vi "有符号24位转32位有符号数.vi"(11 "Registers":u16[](array[numeric])) -> (2 "数字量":i32[](array[numeric]), 3 "工程量":dbl[](array[numeric]))   [LabVIEW 2016, in "采配水.lvlib"]
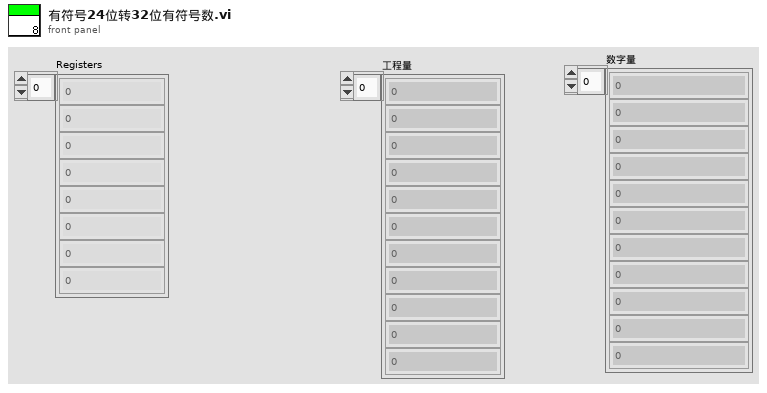
[diagram p1: front panel]
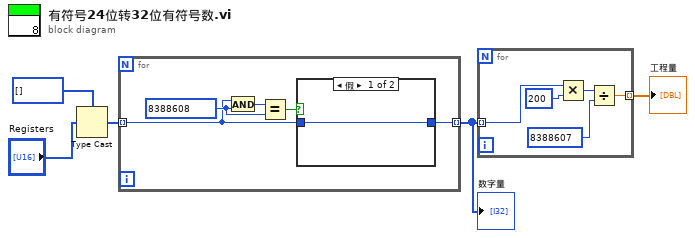
[diagram p0: block diagram]
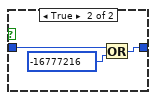
[diagram p2: hidden frame]
diagram:
  n1 = Type Cast(type=i32[] [], x="Registers") -> (*(type *) &x=w3:i32[])
  n2 = for {
    tunnel: w3 -> [w7] mode=indexing
    tunnel: [w6] -> w2 mode=indexing
    w9 = 8388608 ("y")
    n3 = And(x=w7, y=w9) -> (x .and. y?=w10:i32)
    n4 = Equal?(x=w10, y=w9) -> (x = y?=w8:bool)
    n5 = case shown="假" w8 {
      tunnel: w7 -> [w11 w14]
      tunnel: [w11 w12] -> w6
      frame False {
      }
      frame True {
        n6 = Or(x=w14, y=-16777216) -> (x .or. y?=w12:i32)
      }
    }
  }
  "数字量" <- w2
  n7 = for {
    tunnel: w2 -> [w19] mode=indexing
    tunnel: [w15] -> w1 mode=indexing
    n8 = Multiply(x=w19, y=200) -> (x*y=w17:i32)
    n9 = Divide(x=w17, y=8388607) -> (x/y=w15:dbl)
  }
  "工程量" <- w1
